vi "Close.vi"(8 "Error In":errorcluster, 11 "LINX Resource":T1) -> (0 "Error Out":errorcluster, 3 "LINX Resource":T1)   [LabVIEW 2011, in "LVH-LINX.lvlib"]
doc: "Close the connection to the LINX device."
uses:
  LVH-LINX.lvlib
  Private/Type Defs/LINX Ref.ctl
  Private/Type Defs/Platform.ctl
  Private/Type Defs/Interface.ctl
  Private/Device/Type Defs/LINX Device Config.ctl
  Private/Device/Type Defs/TCP Config.ctl
  Private/Type Defs/Device Family.ctl
  Private/Device/Device.lvlib
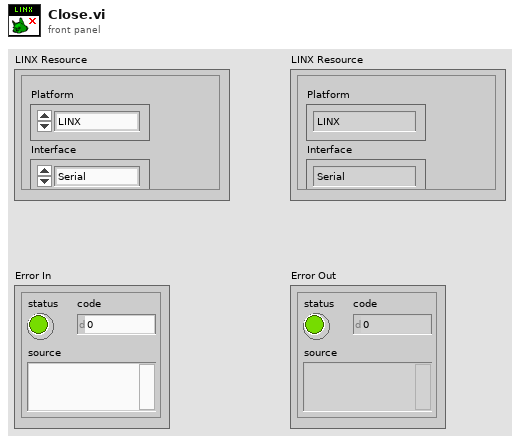
[diagram p1: front panel]
types:
  T1 = typedef "LVH-LINX.lvlib/LINX Ref.ctl" = cluster{"Platform":T2, "Interface":T3, "LINX Device Config":T4}
  T2 = typedef "LVH-LINX.lvlib/Platform.ctl" = enum16{"LINX", "myRIO"}
  T3 = typedef "LVH-LINX.lvlib/Interface.ctl" = enum16{"Serial", "TCP"}
  T4 = typedef "LVH-LINX.lvlib/Device.lvlib/LINX Device Config.ctl" = cluster{"Interface":T3, "COM Port":refnum<visa-resource-name>, "TCP Configuration":T5, "Device Family":T6, "Device ID":u8, "Device Name":string, "TCP Ref":refnum<k5>}
  T5 = typedef "LVH-LINX.lvlib/Device.lvlib/TCP Config.ctl" = cluster{"IP Address":string, "Port":u16}
  T6 = typedef "LVH-LINX.lvlib/Device Family.ctl" = enum8{"National Instruments", "Digilent", "Arduino"}
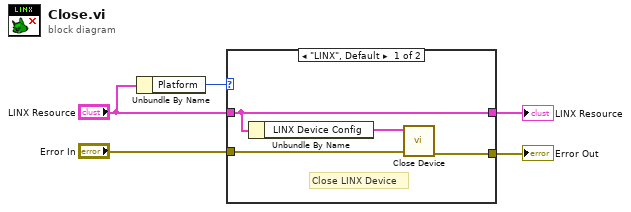
[diagram p0: block diagram]
diagram:
  n1 = Unbundle By Name("LINX Resource") -> ("Platform"=w5:T2)
  n2 = case shown="\"LINX\", Default" w5 {
    tunnel: "LINX Resource" -> [w8 w10]
    tunnel: [w8 w10] -> w3
    tunnel: [w7 w11] -> w2
    tunnel: "Error In" -> [w6 w11]
    frame "LINX", Default {
      # "Close LINX Device"
      n3 = Unbundle By Name(w8) -> ("LINX Device Config"=w9:T4)
      n4 = call "Close Device.vi"("Error In"=w6, "LINX Device Config"=w9) -> ("Error Out"=w7:errorcluster)  [unwired: 8 in, 1 out]
    }
    frame "myRIO" {
      # "Close myRIO"
    }
  }
  "Error Out" <- w2
  "LINX Resource" <- w3
